vi "Get First Serial Port.vi"(7 "Error In":errorcluster) -> (4 "PS Comm Port":refnum<visa-resource-name>, 15 "Error Out":errorcluster)   [LabVIEW 2025]
doc: "Author: Scott Hannahs <sth@magnet.fsu.edu>\n\nThis software is licensed for use under the “MIT License\"\nCopyright (c) 2025 Scott Hannahs, sth@sth@magnet.sthnet.net\n\nPermission is hereby granted, free of charge, to any person obtaining a copy of this software and associated documentation files (the \"Software\"), to deal in the Software without restriction, including without limitation the rights to use, copy, modify, merge, publish, distribute, sublicense, and/or sell copies of the Software, and to permit persons to whom the Software is furnished to do so, subject to the following conditions: The above copyright notice and this permission notice shall be included in all copies or substantial portions of the Software.\n\nTHE SOFTWARE IS PROVIDED \"AS IS\", WITHOUT WARRANTY OF ANY KIND, EXPRESS OR IMPLIED, INCLUDING BUT NOT LIMITED TO THE WARRANTIES OF MERCHANTABILITY, FITNESS FOR A PARTICULAR PURPOSE AND NONINFRINGEMENT. IN NO EVENT SHALL THE AUTHORS OR COPYRIGHT HOLDERS BE LIABLE FOR ANY CLAIM, DAMAGES OR OTHER LIABILITY, WHETHER IN AN ACTION OF CONTRACT, TORT OR OTHERWISE, ARISING FROM, OUT OF OR IN CONNECTION WITH THE SOFTWARE OR THE USE OR OTHER DEALINGS IN THE SOFTWARE."
uses:
  PS Comm Globals.vi
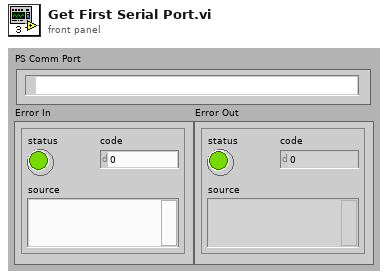
[diagram p1: front panel]
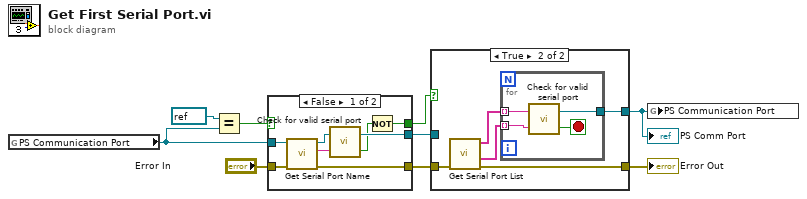
[diagram p0: block diagram]
diagram:
  n1 = global read "PS Comm Globals.vi" "PS Communication Port"() -> (w7:refnum<visa-resource-name>)
  n2 = Equal?(x=refnum<visa-resource-name> refnum ("y"), y=w7) -> (x = y?=w8:bool)
  n3 = case shown="False" w8 {
    selector: w8 -> [_ w20]
    tunnel: [w17 w20] -> w6
    tunnel: w7 -> [w16 w19]
    tunnel: [w15 w19] -> w5
    tunnel: "Error In" -> [w11 w18]
    tunnel: [w10 w18] -> w1
    frame False {
      n4 = call "Get Serial Port Name.vi"("Error In"=w11, "PS Communication Port In"=w16) -> ("Error Out"=w10:errorcluster, "Serial Port Name"=w13:string, "PS Communication Port Out"=w14:refnum<visa-resource-name>)  [unwired: 3 in]
      n5 = call "Check for valid serial port.vi"("Serial Port Name"=w13, "PS Communication Port In"=w14) -> ("Valid Serial Port"=w12:bool, "PS Communication Port out"=w15:refnum<visa-resource-name>)
      n6 = Not(x=w12) -> (.not. x?=w17:bool)
    }
    frame True {
    }
  }
  n7 = case shown="True" w6 {
    tunnel: w5 -> [w22 _]
    tunnel: [w22 w27] -> w4
    tunnel: [w21 w24] -> w2
    tunnel: w1 -> [w21 w23]
    frame False {
    }
    frame True {
      n8 = call "Get Serial Port List.vi"("error in (no error)"=w23) -> ("error out"=w24:errorcluster, "Port Names"=w26:string[], "VISA Name"=w25:string[])  [unwired: 6 in, 2 out]
      n9 = for {
        tunnel: [w30] -> w27
        tunnel: w25 -> [w31] mode=indexing
        tunnel: w26 -> [w29] mode=indexing
        stop <- w28 stop-if-true
        n10 = call "Check for valid serial port.vi"("Serial Port Name"=w29, "PS Communication Port In"=w31) -> ("Valid Serial Port"=w28:bool, "PS Communication Port out"=w30:refnum<visa-resource-name>)
      }
    }
  }
  "PS Comm Port" <- w4
  "Error Out" <- w2
  n11 = global write "PS Comm Globals.vi" "PS Communication Port"(w4) -> ()
